vi "ReadCompoundArithmetic.vi"(1 "reference":refnum<vi>) -> (0 "CompoundArithmetic":T6)   [LabVIEW 2013]
uses:
  <vilib>/Utility/miscctls.llb/LVBoundsTypeDef.ctl
  <vilib>/Utility/miscctls.llb/LVPositionTypeDef.ctl
  <vilib>/Utility/miscctls.llb/LVRectTypeDef.ctl
  <vilib>/Utility/miscctls.llb/LVBreakpointStatusEnum.ctl
  <vilib>/picture/picture.llb/imagedata.ctl
panel:
  out "error out 24":errorcluster
  out "error out 23":errorcluster
  out "error out 22":errorcluster
  out "error out 21":errorcluster
  out "error out 20":errorcluster
  out "error out 19":errorcluster
  out "error out 18":errorcluster
  out "error out 17":errorcluster
  out "error out 16":errorcluster
  out "error out 15":errorcluster
  out "error out 14":errorcluster
  out "error out 13":errorcluster
  out "error out 12":errorcluster
  out "error out 11":errorcluster
  out "error out 10":errorcluster
  out "error out 9":errorcluster
  out "error out 8":errorcluster
  out "error out 7":errorcluster
  out "error out 6":errorcluster
  out "error out 5":errorcluster
  out "error out 4":errorcluster
  out "error out 3":errorcluster
  out "error out 2":errorcluster
  out "error out":errorcluster
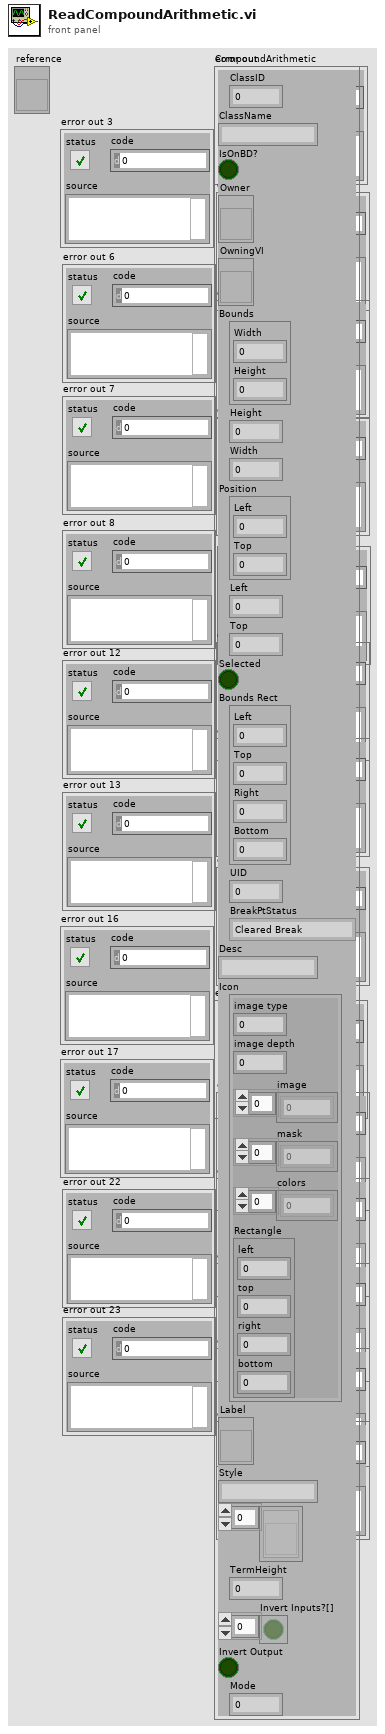
[diagram p1: front panel]
types:
  T1 = typedef "LVBoundsTypeDef.ctl" = cluster{"Width":u32, "Height":u32}
  T2 = typedef "LVPositionTypeDef.ctl" = cluster{"Left":i32, "Top":i32}
  T3 = typedef "LVRectTypeDef.ctl" = cluster{"Left":i16, "Top":i16, "Right":i16, "Bottom":i16}
  T4 = typedef "LVBreakpointStatusEnum.ctl" = enum8{"Cleared Break", "Enabled Break", "Disabled Break"}
  T5 = typedef "imagedata.ctl" = cluster{"image type":i32, "image depth":i32, "image":u8[], "mask":u8[], "colors":u32[], "Rectangle":cluster{"left":i16, "top":i16, "right":i16, "bottom":i16}}
  T6 = cluster{"ClassID":u32, "ClassName":string, "IsOnBD?":bool, "Owner":refnum<vi>, "OwningVI":refnum<vi>, "Bounds":T1, "Height":u32, "Width":u32, "Position":T2, "Left":i32, "Top":i32, "Selected":bool, "Bounds Rect":T3, "UID":i32, "BreakPtStatus":T4, "Desc":string, "Icon":T5, "Label":refnum<vi>, "Style":string, "Terms[]":refnum<vi>[], "TermHeight":i32, "Invert Inputs?[]":bool[], "Invert Output":bool, "Mode":u32}
  T7 = cluster{"ClassID":u32, "ClassName":string, "IsOnBD?":bool, "Owner":refnum<vi>, "OwningVI":refnum<vi>, "Bounds":T1, "Height":u32, "Width":u32, "Position":T2, "Left":i32, "Top":i32, "Selected":bool, "Bounds Rect":T3, "UID":i32, "BreakPtStatus":T4, "Desc":string, "Icon":T5, "Label":refnum<vi>, "Style":string, refnum<vi>[], "TermHeight":i32, "Invert Inputs?[]":bool[], "Invert Output":bool, "Mode":u32}
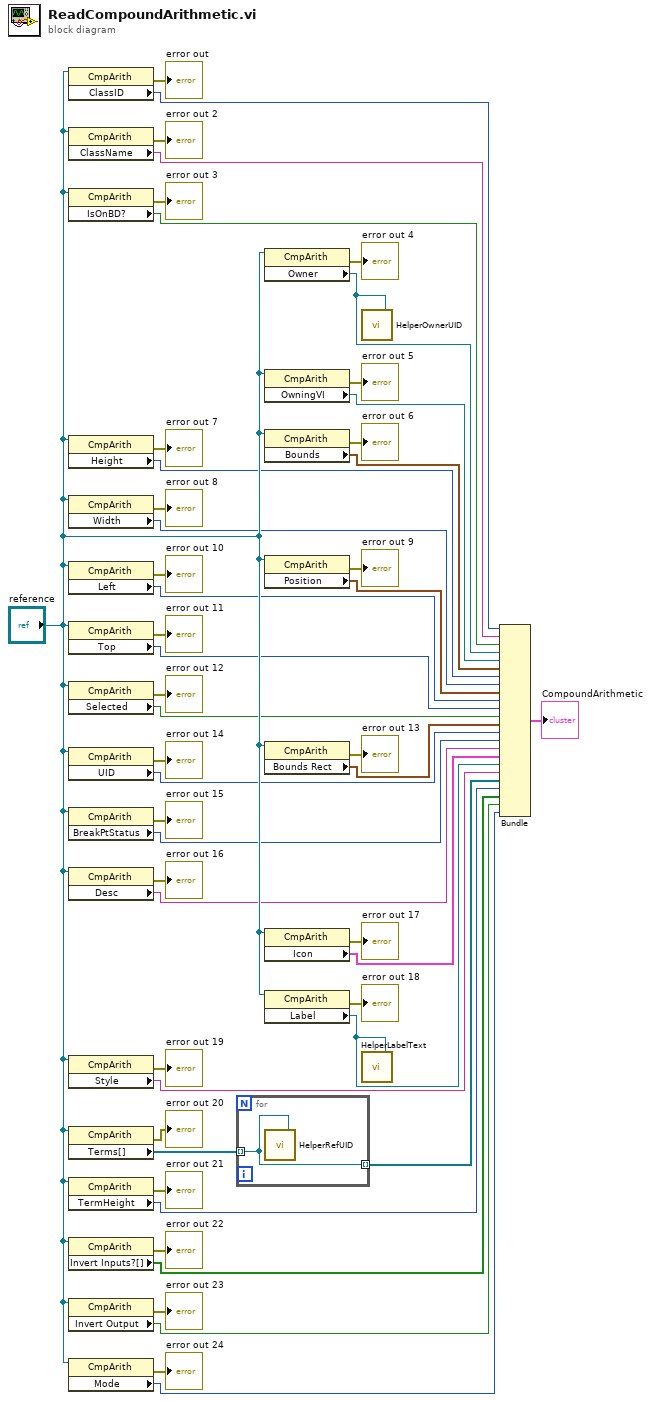
[diagram p0: block diagram]
diagram:
  n1 = property class="CmpArith"(reference="reference") -> (error out=→"error out":errorcluster, "ClassID"=w49:u32)  [unwired: 1 in, 1 out]
  n2 = property class="CmpArith"(reference="reference") -> (error out=→"error out 2":errorcluster, "ClassName"=w47:string)  [unwired: 1 in, 1 out]
  n3 = property class="CmpArith"(reference="reference") -> (error out=→"error out 3":errorcluster, "IsOnBD?"=w45:bool)  [unwired: 1 in, 1 out]
  n4 = property class="CmpArith"(reference="reference") -> (error out=→"error out 7":errorcluster, "Height"=w37:u32)  [unwired: 1 in, 1 out]
  n5 = property class="CmpArith"(reference="reference") -> (error out=→"error out 8":errorcluster, "Width"=w35:u32)  [unwired: 1 in, 1 out]
  n6 = property class="CmpArith"(reference="reference") -> (error out=→"error out 10":errorcluster, "Left"=w31:i32)  [unwired: 1 in, 1 out]
  n7 = property class="CmpArith"(reference="reference") -> (error out=→"error out 11":errorcluster, "Top"=w29:i32)  [unwired: 1 in, 1 out]
  n8 = property class="CmpArith"(reference="reference") -> (error out=→"error out 12":errorcluster, "Selected"=w27:bool)  [unwired: 1 in, 1 out]
  n9 = property class="CmpArith"(reference="reference") -> (error out=→"error out 14":errorcluster, "UID"=w23:i32)  [unwired: 1 in, 1 out]
  n10 = property class="CmpArith"(reference="reference") -> (error out=→"error out 15":errorcluster, "BreakPtStatus"=w21:T4)  [unwired: 1 in, 1 out]
  n11 = property class="CmpArith"(reference="reference") -> (error out=→"error out 16":errorcluster, "Desc"=w19:string)  [unwired: 1 in, 1 out]
  n12 = property class="CmpArith"(reference="reference") -> (error out=→"error out 19":errorcluster, "Style"=w13:string)  [unwired: 1 in, 1 out]
  n13 = property class="CmpArith"(reference="reference") -> (error out=→"error out 20":errorcluster, "Terms[]"=w11:refnum<vi>[])  [unwired: 1 in, 1 out]
  n14 = property class="CmpArith"(reference="reference") -> (error out=→"error out 21":errorcluster, "TermHeight"=w8:i32)  [unwired: 1 in, 1 out]
  n15 = property class="CmpArith"(reference="reference") -> (error out=→"error out 22":errorcluster, "Invert Inputs?[]"=w6:bool[])  [unwired: 1 in, 1 out]
  n16 = property class="CmpArith"(reference="reference") -> (error out=→"error out 23":errorcluster, "Invert Output"=w4:bool)  [unwired: 1 in, 1 out]
  n17 = property class="CmpArith"(reference="reference") -> (error out=→"error out 24":errorcluster, "Mode"=w2:u32)  [unwired: 1 in, 1 out]
  n18 = for {
    tunnel: w11 -> [w52] mode=indexing
    tunnel: [w52] -> w10 mode=indexing
    n19 = call "HelperRefUID.vi"("Text in"=w52) -> ()  [unwired: 1 out]
  }
  n20 = property class="CmpArith"(reference="reference") -> (error out=→"error out 4":errorcluster, "Owner"=w43:refnum<vi>)  [unwired: 1 in, 1 out]
  n21 = property class="CmpArith"(reference="reference") -> (error out=→"error out 5":errorcluster, "OwningVI"=w41:refnum<vi>)  [unwired: 1 in, 1 out]
  n22 = property class="CmpArith"(reference="reference") -> (error out=→"error out 6":errorcluster, "Bounds"=w39:T1)  [unwired: 1 in, 1 out]
  n23 = property class="CmpArith"(reference="reference") -> (error out=→"error out 9":errorcluster, "Position"=w33:T2)  [unwired: 1 in, 1 out]
  n24 = property class="CmpArith"(reference="reference") -> (error out=→"error out 13":errorcluster, "Bounds Rect"=w25:T3)  [unwired: 1 in, 1 out]
  n25 = property class="CmpArith"(reference="reference") -> (error out=→"error out 17":errorcluster, "Icon"=w17:T5)  [unwired: 1 in, 1 out]
  n26 = property class="CmpArith"(reference="reference") -> (error out=→"error out 18":errorcluster, "Label"=w15:refnum<vi>)  [unwired: 1 in, 1 out]
  n27 = call "HelperOwnerUID.vi"("Generic in"=w43) -> ()  [unwired: 1 out]
  n28 = call "HelperLabelText.vi"("Text in"=w15) -> ()  [unwired: 1 out]
  n29 = Bundle("ClassID"=w49, "ClassName"=w47, "IsOnBD?"=w45, "Owner"=w43, "OwningVI"=w41, "Bounds"=w39, "Height"=w37, "Width"=w35, "Position"=w33, "Left"=w31, "Top"=w29, "Selected"=w27, "Bounds Rect"=w25, "UID"=w23, "BreakPtStatus"=w21, "Desc"=w19, "Icon"=w17, "Label"=w15, "Style"=w13, w10, "TermHeight"=w8, "Invert Inputs?[]"=w6, "Invert Output"=w4, "Mode"=w2) -> (→"CompoundArithmetic":T7)  [unwired: 1 in]
